vi "Set Config.vi"(8 "error in (no error)":errorcluster, 10 "Config":T1[](array[typedef]), 11 "DeployResource in":refnum<class "Resource.lvclass">) -> (0 "error out":errorcluster, 3 "DeployResource out":refnum<class "Resource.lvclass">)   [LabVIEW 2020, in "PicoG-Core.lvlib" / "Resource.lvclass"]
uses:
  Resource.lvclass
  Resource.lvclass/Resource.ctl
  Config Item.ctl
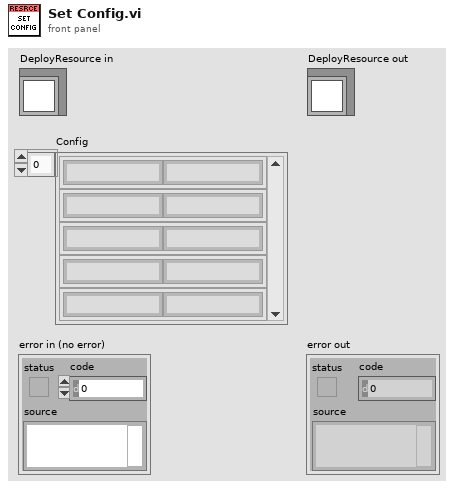
[diagram p1: front panel]
types:
  T1 = typedef "PicoG-Core.lvlib/Resource.lvclass/Config Item.ctl" = cluster{"Key":string, "Value":string}
  T2 = typedef "PicoG-Core.lvlib/Resource.lvclass/Ref Data.ctl" = cluster{"Config":map{string, string}, "Stream":refnum<class "Stream.lvclass">}
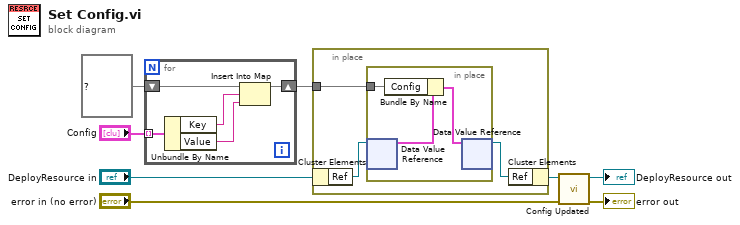
[diagram p0: block diagram]
diagram:
  n1 = for {
    tunnel: "Config" -> [w13] mode=indexing
    shift-right: [w9] -> w1
    shift-left: map{string, string} {} ("map") -> [w12]
    n2 = Unbundle By Name(w13) -> ("Key"=w11:string, "Value"=w10:string)
    n3 = Insert Into Map(map in=w12, key=w11, value=w10) -> (map out=w9:map{string, string})  [unwired: 2 out]
  }
  n4 = in-place {
    in-place-border: w1 -> [w14]
    n5 = in-place-cluster #1("DeployResource in") -> ("Ref"=w16:refnum<data-value>)
    n6 = in-place {
      in-place-border: w14 -> [w18]
      n7 = in-place-dvr #2(w16) -> (w19:T2)  [unwired: 1 out]
      n8 = Bundle By Name(cluster=w19, "Config"=w18) -> (w17:T2)
      n9 = in-place-dvr #2(w17) -> (w15:refnum<data-value>)  [unwired: 1 out]
    }
    n10 = in-place-cluster #1("Ref"=w15) -> (w2:refnum<class "Resource.lvclass">)
  }
  n11 = call-dynamic "Config Updated.vi"("error in (no error)"="error in (no error)", "Resource in"=w2) -> ("error out"=→"error out":errorcluster, "Resource out"=→"DeployResource out":refnum<class "Resource.lvclass">)  [unwired: 8 in]
